vi "OFF_Polarity_Channel_Manual.vi"(5 "CH_ON:0/OFF:1":u16, 7 "Mode":u16(ring)=1 items=["Tx"=1, "Rx"=2], 8 "error in":errorcluster, 11 "TCPIPin":T1={"address"="192.168.100.111", "remote port or service name"=5025, "timeout ms (60000)"=10000}) -> (0 "error out":errorcluster, 1 "OK?":bool, 3 "TCPIPout":T1={"address"="192.168.100.111", "remote port or service name"=5025, "timeout ms (60000)"=10000})   [LabVIEW 2020]
panel:
  in  "x":i32
  in  "Polarity":u16(ring) items=["V", "H"]
  out "Array":string[][](array[string])
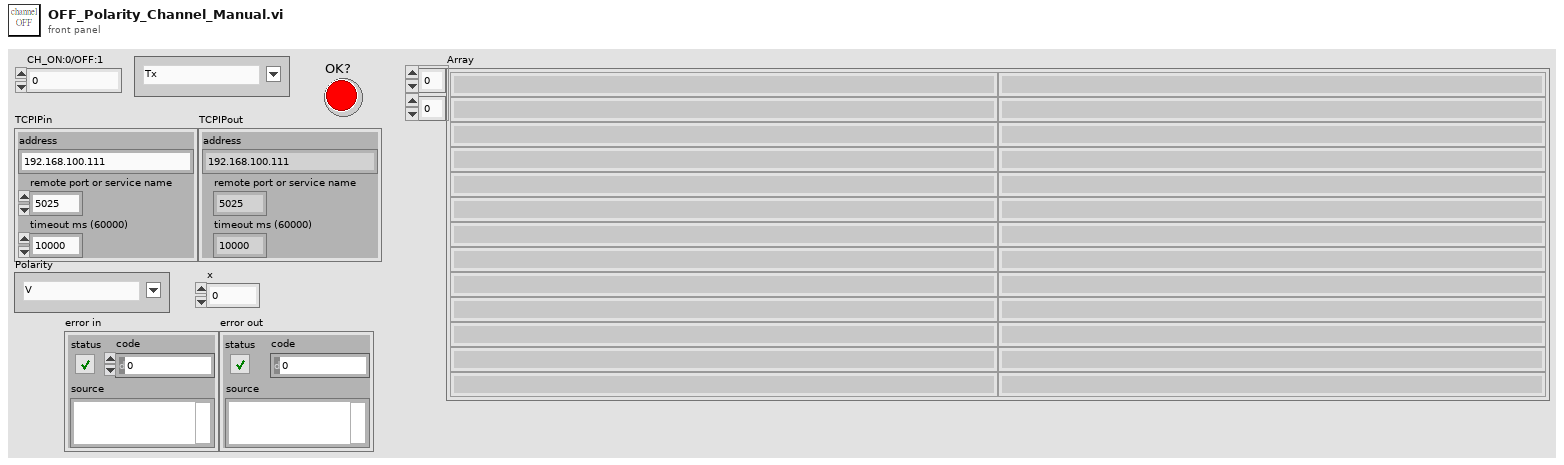
[diagram p1: front panel]
types:
  T1 = cluster{"address":string, "remote port or service name":u16, "timeout ms (60000)":i32}
  T2 = cluster{"Mode":u16, "Polarity":u16, "CH_ON/OFF":u16, "Channel":i32, "Gain":i32, "Phase":i32}
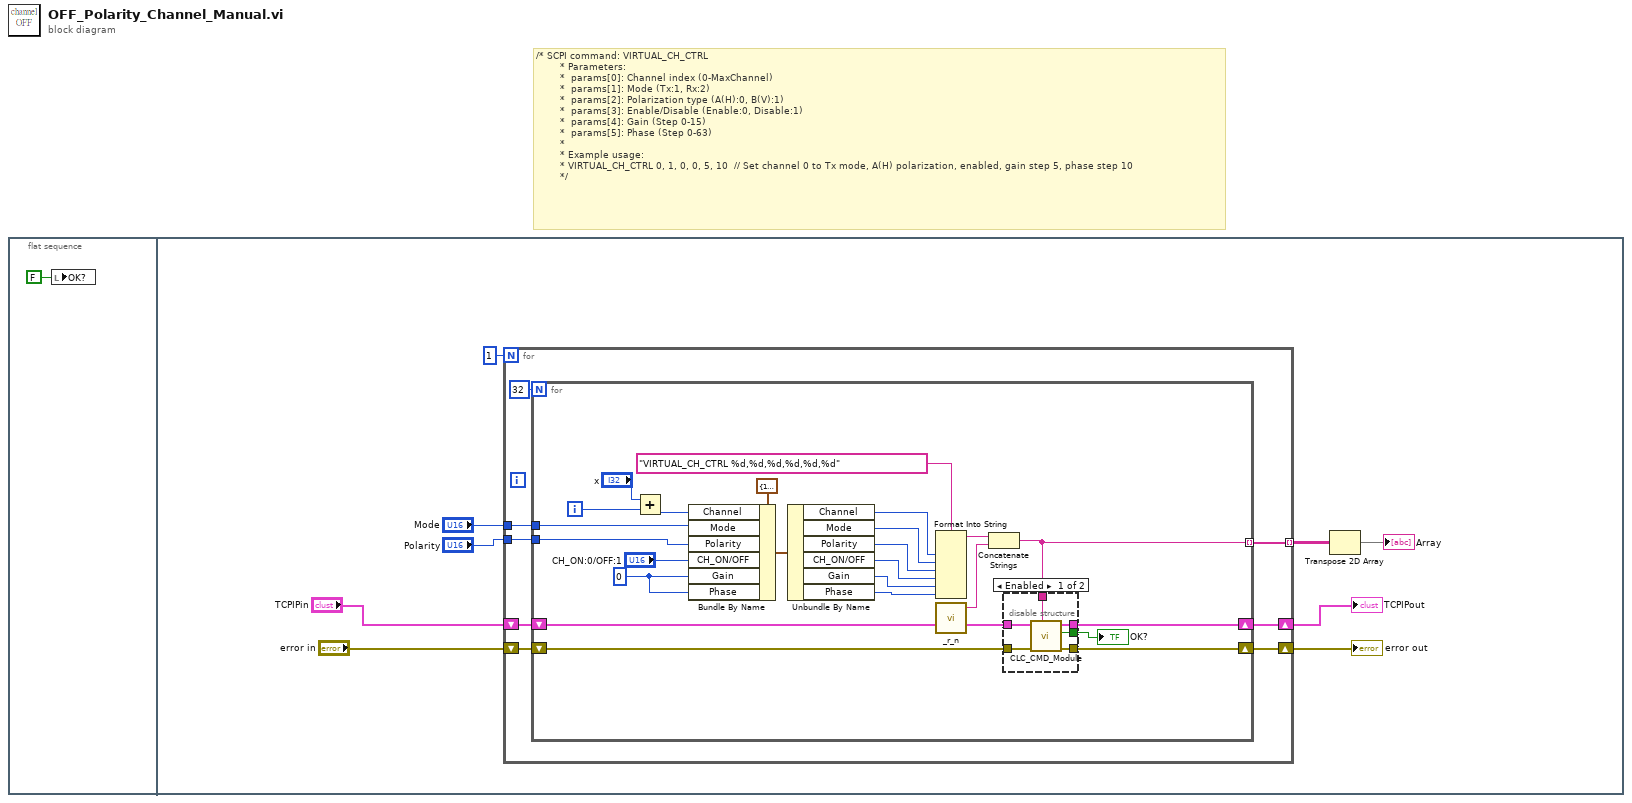
[diagram p0: block diagram]
diagram:
  # "/* SCPI command: VIRTUAL_CH_CTRL\n        * Parameters:\n        *  params[0]: Channel index (0-MaxChannel)\n        *  params[1]: Mode (Tx:1, Rx:2)\n        *  params[2]: Polarization type (A(H):0, B(V):1)\n        *  params[3]: Enable/Disable (Enable:0, Disable:1)\n        *  params[4]: Gain (Step 0-15)\n        *  params[5]: Phase (Step 0-63)\n        * \n        * Example usage:\n        * VIRTUAL_CH_CTRL 0, 1, 0, 0, 5, 10  // Set channel 0 to Tx mode, A(H) polarization, enabled, gain step 5, phase step 10\n        */"
  n1 = flat-sequence {
    frame #0 {
      n2 = local write "OK?"(FALSE ("OK?")) -> ()
    }
    frame #1 {
      n3 = for {
        N: 1 -> [_]
        shift-right: [w17] -> w9
        shift-left: "TCPIPin" -> [w18]
        shift-right: [w15] -> w7
        shift-left: "error in" -> [w16]
        tunnel: "Mode" -> [w13]
        tunnel: [w12] -> w4 mode=indexing
        tunnel: "Polarity" -> [w11]
        n4 = for {
          N: 32 -> [_]
          shift-right: [w41] -> w17
          shift-left: w18 -> [w42]
          shift-right: [w39] -> w15
          shift-left: w16 -> [w40]
          tunnel: w13 -> [w27]
          tunnel: [w23] -> w12 mode=indexing
          tunnel: w11 -> [w21]
          i -> [w25]
          w24 = 0 ("Gain")
          n5 = Add(x="x", y=w25) -> (x+y=w20:i32)
          n6 = Bundle By Name(cluster=T2 {"Mode"=1, "Polarity"=1, "CH_ON/OFF"=1, "Channel"=0, "Gain"=0, "Phase"=0} ("Channel params"), "Channel"=w20, "Mode"=w27, "Polarity"=w21, "CH_ON/OFF"="CH_ON:0/OFF:1", "Gain"=w24, "Phase"=w24) -> (w28:T2)
          n7 = Unbundle By Name(w28) -> ("Channel"=w33:i32, "Mode"=w34:u16, "Polarity"=w35:u16, "CH_ON/OFF"=w36:u16, "Gain"=w37:i32, "Phase"=w38:i32)
          n8 = Format Into String(format string="VIRTUAL_CH_CTRL %d,%d,%d,%d,%d,%d" ("data in"), w33, w34, w35, w36, w37, w38) -> (resulting string=w31:string)  [unwired: 2 in, 1 out]
          n9 = call "_r_n.vi"() -> ("command"=w32:string)  [unwired: 5 in]
          n10 = Concatenate Strings(w31, w32) -> (w23:string)
          n11 = disable-structure shown="Enabled" {
            disable-tunnel: w42 -> [w48 w50]
            disable-tunnel: [w47 w50] -> w41
            disable-tunnel: w40 -> [w46 w49]
            disable-tunnel: [w45 w49] -> w39
            disable-tunnel: w23 -> [w44 _]
            disable-tunnel: [w43 _] -> w26
            frame Enabled {
              n12 = call "CLC_CMD_Module.vi"("CMD in"=w44, "error in"=w46, "TCPIPin"=w48) -> ("error out"=w45:errorcluster, "OK?"=w43:bool, "TCPIPout"=w47:T1)  [unwired: 6 in]
            }
            frame Disabled {
            }
          }
          "OK?" <- w26
        }
      }
      "TCPIPout" <- w9
      "error out" <- w7
      n13 = Transpose 2D Array(2D array=w4) -> (transposed array=→"Array":string[][])
    }
  }
